vi "nanocal -- nuclear schottky goodness gradient.vi"(0 "zeta":dbl(slide)=0.23496699999999998 min=0.0 max=0.3 step=1e-06 scale=0.01..10.0 scale format="%#_3p", 1 "T1":dbl(slide)=0.26762 min=0.0 max=0.3 step=1e-06 scale=0.001..10.0 scale format="%#_3p", 2 "tauS":dbl(slide)=0.24445899999999998 min=0.0 max=0.3 step=1e-06 scale=0.001..10.0 scale format="%#_3p", 3 "tauN":dbl(slide)=2.349673 min=0.0 max=0.3 step=1e-06 scale=0.001..10.0 scale format="%#_3p", 4 "tauC":dbl(slide)=0.0059759999999999995 min=0.0 max=0.3 step=1e-06 scale=0.001..10.0 scale format="%#_3p", 5 "kappa0":dbl(slide)=5.58e-10 min=0.0 max=0.3 step=1e-12 scale=1e-10..1e-06 scale format="%#_3p", 6 "action":T1, 7 "Freq  (rad/sec)":dbl[](array[numeric])=[32012.991918577427, 32390.261658505893, 32466.39798177853, 32499.14340521798, 32517.39286113775, 32529.046092051318, 32537.14525712326, 32543.111142615544, 32547.696343954158, 32551.33675949651, 32554.302325209504, 32556.769142360055, 32558.856995237307, 32560.650202739795, 32562.209843476354, 32563.58125099723, 32564.7987833122, 32565.88895894197, 32566.872575330308, 32567.766175404246, 32568.583086316496, 32569.334166794306, 32570.02835688638, 32570.673085530187, 32571.274580490695, 32571.838104118455, 32572.36813539066, 32572.868514009202, 32573.342552524307, 32573.793126289274, 32574.222746575288, 32574.633618125405, 32575.027687968828, 32575.40668442971, 32575.772149741057, 32576.12546690325, 32576.467883345118, 32576.800529469096, 32577.124435064776, 32577.440543590797, 32577.749724325146, 32578.052781957467, 32578.35046682089, 32578.643482565894, 32578.932492128843, 32579.218126471686, 32579.500987779396, 32579.781656707495, 32580.06069600583, 32580.338656060805, 32580.616078519142, 32580.89350097748, 32581.171461032456, 32581.45050033079, 32581.73116925889, 32582.0140305666, 32582.29966469628, 32582.58867447239, 32582.88169000423, 32583.179375080817, 32583.48243271314, 32583.791613234323, 32584.10772197351, 32584.43162756919, 32584.764273480003, 32585.106690135035, 32585.460007297228, 32585.825472395412, 32586.204468856296, 32586.59853891288, 32587.009410462997, 32587.439030535847, 32587.889604513977, 32588.363642815923, 32588.86402143446, 32589.39405291983, 32589.957576334426, 32590.559071508098, 32591.203800151903, 32591.897990030815, 32592.64907072179, 32593.46598163404, 32594.359581707977, 32595.343197883154, 32596.433373726086, 32597.650906041054, 32599.022313348767, 32600.58195429849, 32602.375161800977, 32604.46301467823, 32606.929831615616, 32609.895397541775, 32613.535812870963, 32618.12101442274, 32624.086899701866, 32632.186064986967, 32643.839295900536, 32662.088751820305, 32694.834175046595, 32770.97049853239], 8 "dlogstep":dbl=0.0001 format="%#_13g", 9 "Voltage out (V)":cdb[](array[numeric])=[1.7183506006211996e-05-0.0001154032788780638i, 1.7124360968751133e-05-0.0001154114779288915i, 1.7049104347380084e-05-0.00011541542942613611i, 1.700437896335042e-05-0.00011541749156201827i, 1.6984579723285106e-05-0.00011542204741013496i, 1.702277369054923e-05-0.00011543195548892015i, 1.713094025845651e-05-0.00011543928112855599i, 1.734249707866828e-05-0.00011543960094139092i, 1.768320429215342e-05-0.0001154245402225022i, 1.8195281152538477e-05-0.00011538335923575508i, 1.8917228661806973e-05-0.00011530288392402138i, 1.9897834564883332e-05-0.00011516640933089982i, 2.154104046962704e-05-0.0001148906117047364i, 2.3247799321765792e-05-0.00011455940834964969i, 2.5364678450551808e-05-0.00011410149936074356i, 2.8645788781885885e-05-0.00011331572480450341i, 3.204749554800641e-05-0.00011242961468546203i, 3.783559691555022e-05-0.00011080033368711338i, 4.245015867332296e-05-0.00010941815048749576i, 4.909131821431355e-05-0.0001073312840925185i, 5.511821898441184e-05-0.00010535829212367013i, 6.178843506022867e-05-0.00010310289174359778i, 7.1079604965352e-05-9.985157907779013e-05i, 7.922304381453334e-05-9.690255343156676e-05i, 8.814778883893872e-05-9.35627973091444e-05i, 9.806709148886077e-05-8.971246458508318e-05i, 0.00011119043245647465-8.437841897470898e-05i, 0.00012253184919712196-7.953180105990741e-05i, 0.00013777724317049346-7.26422052575784e-05i, 0.0001508081004573332-6.638511645494567e-05i, 0.00016547294918783876-5.890291826790314e-05i, 0.00018003847596605868-5.097295421607585e-05i, 0.00019518361086534857-4.2160672625888326e-05i, 0.00021134179818259658-3.207632261667366e-05i, 0.0002372041782935464-1.434566976209705e-05i, 0.00025518143132024254-7.65423157605567e-07i, 0.0002835129702467886+2.297908707067173e-05i, 0.0003060118087631287+4.414715126576145e-05i, 0.00032860772064336976+6.780161699354136e-05i, 0.0003492674091322389+9.188627597766353e-05i, 0.00037498324855458583+0.0001258445655672888i, 0.00040021078021115026+0.00016463936720210011i, 0.00041969942568205823+0.0001996255883353531i, 0.00044367338947118773+0.00025154867300893595i, 0.0004634793607238068+0.0003068834938295352i, 0.00047921028781215815+0.00036805191402776324i, 0.0004880906353641744+0.00042166295770603194i, 0.0004932212623741357+0.0004947057496862386i, 0.000491476456593048+0.0005562791342814882i, 0.000480893803992059+0.0006363872629062725i, 0.0004535995818650303+0.0007373086546111893i, 0.000417087772881063+0.0008226852134031236i, 0.0003564148692854789+0.0009214817173403453i, 0.0003049201646356487+0.0009841224100520793i, 0.00021260191240459413+0.0010684135492785532i, 0.00011714858948470126+0.001130293664798013i, 1.675457544365132e-05+0.0011752384955043165i, -6.8674075405897e-05+0.0012001399159748158i, -0.000156473047607305+0.0012143601357779102i, -0.00026709373934749337+0.0012167952520739987i, -0.0003544271565676041+0.001206585218500233i, -0.00047937600197311275+0.0011721904461218277i, -0.0006086290582260493+0.0011080263068835828i, -0.0007031877411848573+0.0010369948237613604i, -0.0007564526901441745+0.0009845652865779295i, -0.000802489180995596+0.0009292050493656664i, -0.0008414596018105983+0.0008721985101652608i, -0.0008809346482248761+0.0008000538120167723i, -0.0009073902840241921+0.0007382113118499092i, -0.0009264953054508651+0.000680980624166274i, -0.0009405659412141811+0.0006247883223244968i, -0.000951649722530156+0.0005564170049287236i, -0.0009557485581057351+0.0005027508202624884i, -0.0009558464741053665+0.0004515634249715623i, -0.0009509110176922098+0.0003899637122391104i, -0.0009411315169847015+0.00033238768338539245i, -0.0009303400913929496+0.0002890952314710416i, -0.0009171113529290538+0.00024772942260094455i, -0.0009022111527275027+0.00020961974320628598i, -0.0008813746494947608+0.00016554205395646727i, -0.0008581837971946129+0.00012481593212717478i, -0.0008372063466683705+9.328565348151487e-05i, -0.0008165626610594428+6.595676342721183e-05i, -0.0007901155435838691+3.51376371228606e-05i, -0.0007682834352800848+1.2585785624721776e-05i, -0.000746231015527196-7.956667433689733e-06i, -0.0007238798463130141-2.6771164006128246e-05i, -0.0007015567569177018-4.3779400880525094e-05i, -0.000679301954671598-5.9154880569231366e-05i, -0.0006572001413831251-7.301304884663801e-05i, -0.000629855254567978-8.838260380910578e-05i, -0.0006083942229188815-9.917719243438264e-05i, -0.0005768631156754208-0.00011317657292622015i, -0.0005562177438951648-0.00012121832857134644i, -0.0005359092039599222-0.00012831021292074535i, -0.0005145186443378148-0.00013494179211461784i, -0.0004951602053444319-0.00014023403510992087i, -0.00047624970229075174-0.00014478034103386663i, -0.0004577401041527736-0.00014865456703421655i, -0.00043519037796120065-0.00015262867452433312i], 10 "nymber of steps":i32=11) -> (14 "derivative":dbl format="%0.4f", 17 "goodness":dbl, 18 "log10goodness":dbl)   [LabVIEW 2020]
uses:
  3-lorentzian-heat-response action.ctl
  3-lorentzian-heat-response.vi
  3-lorentzian-heat-response.vi/142dd4c5-f9ed-c64b-bc14-a88e3e2c450a.vi
  <vilib>/Analysis/polynomials.llb/Multiply Polynomials.vi
  <vilib>/Analysis/polynomials.llb/Multiply Polynomials (DBL).vi
  <vilib>/Analysis/polynomials.llb/Polynomial Roots.vi
  <vilib>/Analysis/polynomials.llb/Polynomial Roots (DBL).vi
  <vilib>/Comparison/Less/Less Functor/Less Functor.lvclass
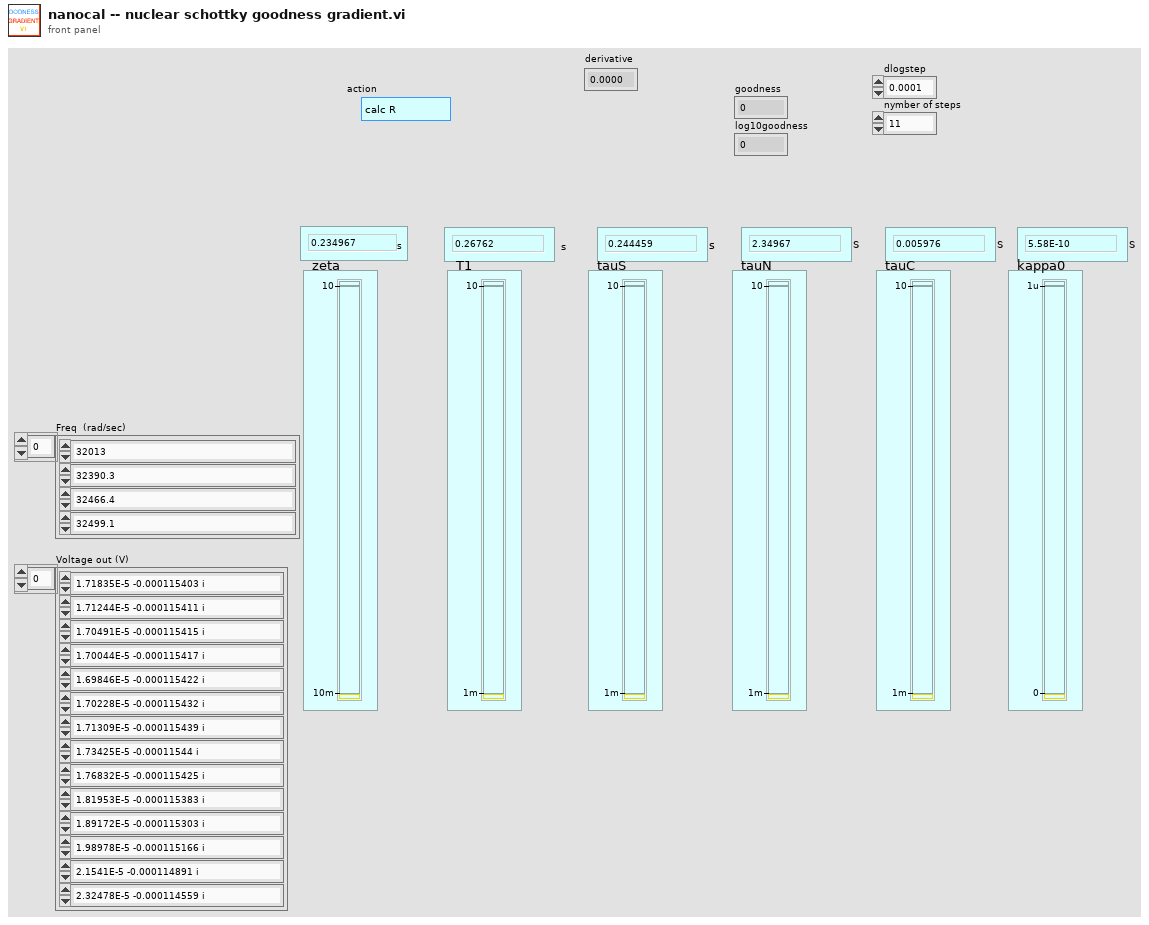
[diagram p1: front panel]
types:
  T1 = typedef "3-lorentzian-heat-response action.ctl" = enum16{"calc R", "create string", "calc m1m2m3", "dζ", "dT1", "dτS", "dτN", "dτC", "d-all", "dκ0"}
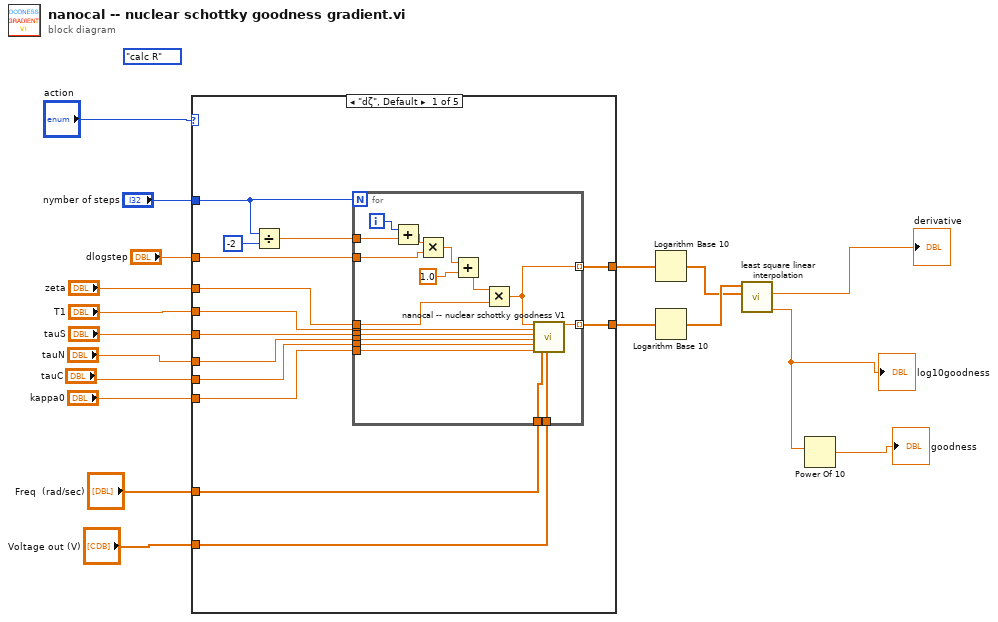
[diagram p0: block diagram]
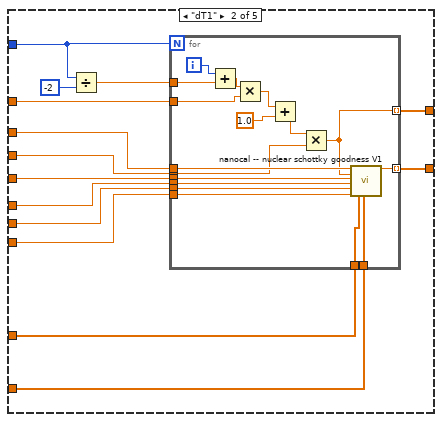
[diagram p2: hidden frame]
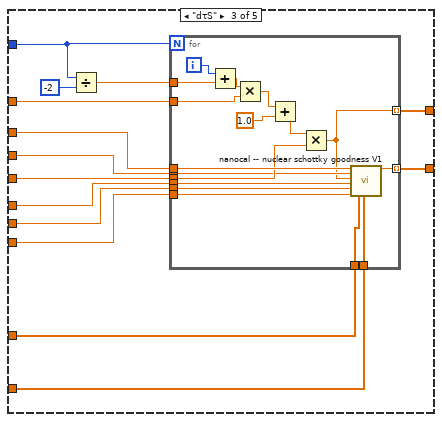
[diagram p3: hidden frame]
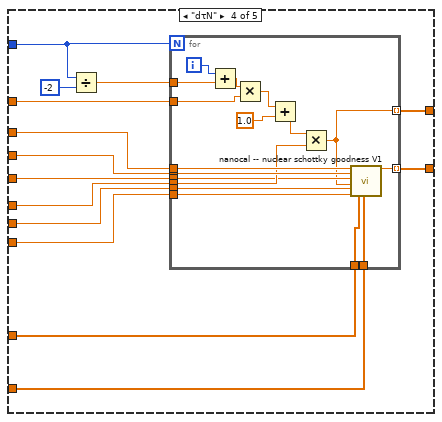
[diagram p4: hidden frame]
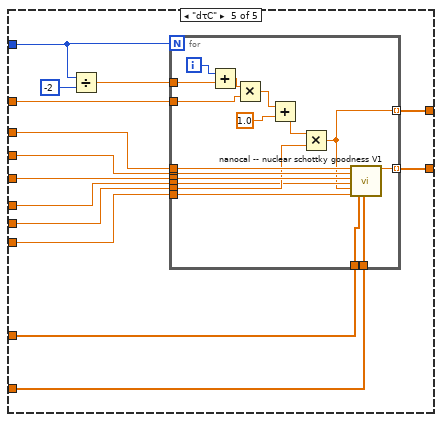
[diagram p5: hidden frame]
diagram:
  (unwired) 3-lorentzian-heat-response_action."calc R" ("action")
  n1 = case shown="\"dζ\", Default" "action" {
    tunnel: "T1" -> [w32 w63 w94 w125 w156]
    tunnel: "tauS" -> [w31 w62 w93 w124 w155]
    tunnel: "tauN" -> [w30 w61 w92 w123 w154]
    tunnel: "tauC" -> [w29 w60 w91 w122 w153]
    tunnel: [w28 w59 w90 w121 w152] -> w9
    tunnel: "Freq  (rad/sec)" -> [w27 w58 w89 w120 w151]
    tunnel: "Voltage out (V)" -> [w26 w57 w88 w119 w150]
    tunnel: "kappa0" -> [w24 w55 w86 w117 w148]
    tunnel: "zeta" -> [w25 w56 w87 w118 w149]
    tunnel: [w19 w50 w81 w112 w143] -> w10
    tunnel: "nymber of steps" -> [w21 w52 w83 w114 w145]
    tunnel: "dlogstep" -> [w20 w51 w82 w113 w144]
    frame "dζ", Default {
      n2 = Divide(x=w21, y=-2) -> (x/y=w22:dbl)
      n3 = for {
        N: w21 -> [_]
        tunnel: w32 -> [w49]
        tunnel: w31 -> [w48]
        tunnel: w30 -> [w47]
        tunnel: w29 -> [w46]
        tunnel: [w45] -> w28 mode=indexing
        tunnel: w27 -> [w44]
        tunnel: w26 -> [w43]
        tunnel: w25 -> [w35]
        tunnel: w24 -> [w42]
        tunnel: w22 -> [w40]
        tunnel: w20 -> [w36]
        tunnel: [w33] -> w19 mode=indexing
        i -> [w41]
        n4 = Add(x=w41, y=w40) -> (x+y=w39:dbl)
        n5 = Multiply(x=w39, y=w36) -> (x*y=w38:dbl)
        n6 = Add(x=w38, y=1.0) -> (x+y=w34:dbl)
        n7 = Multiply(x=w34, y=w35) -> (x*y=w33:dbl)
        n8 = call "nanocal -- nuclear schottky goodness V1.vi"("ζ"=w33, "T1"=w49, "τS"=w48, "τN"=w47, "τC"=w46, "κ0"=w42, "Freq out (rad/sec)"=w44, "Voltage out (V)"=w43) -> ("result"=w45:dbl)  [unwired: 11 in]
      }
    }
    frame "dT1" {
      n9 = Divide(x=w52, y=-2) -> (x/y=w53:dbl)
      n10 = for {
        N: w52 -> [_]
        tunnel: w63 -> [w65]
        tunnel: w62 -> [w80]
        tunnel: w61 -> [w79]
        tunnel: w60 -> [w78]
        tunnel: [w77] -> w59 mode=indexing
        tunnel: w58 -> [w76]
        tunnel: w57 -> [w75]
        tunnel: w56 -> [w66]
        tunnel: w55 -> [w74]
        tunnel: w53 -> [w72]
        tunnel: w51 -> [w68]
        tunnel: [w64] -> w50 mode=indexing
        i -> [w73]
        n11 = Add(x=w73, y=w72) -> (x+y=w71:dbl)
        n12 = Multiply(x=w71, y=w68) -> (x*y=w70:dbl)
        n13 = Add(x=w70, y=1.0) -> (x+y=w67:dbl)
        n14 = Multiply(x=w67, y=w65) -> (x*y=w64:dbl)
        n15 = call "nanocal -- nuclear schottky goodness V1.vi"("ζ"=w66, "T1"=w64, "τS"=w80, "τN"=w79, "τC"=w78, "κ0"=w74, "Freq out (rad/sec)"=w76, "Voltage out (V)"=w75) -> ("result"=w77:dbl)  [unwired: 11 in]
      }
    }
    frame "dτS" {
      n16 = Divide(x=w83, y=-2) -> (x/y=w84:dbl)
      n17 = for {
        N: w83 -> [_]
        tunnel: w94 -> [w96]
        tunnel: w93 -> [w97]
        tunnel: w92 -> [w111]
        tunnel: w91 -> [w110]
        tunnel: [w109] -> w90 mode=indexing
        tunnel: w89 -> [w108]
        tunnel: w88 -> [w107]
        tunnel: w87 -> [w98]
        tunnel: w86 -> [w106]
        tunnel: w84 -> [w104]
        tunnel: w82 -> [w100]
        tunnel: [w95] -> w81 mode=indexing
        i -> [w105]
        n18 = Add(x=w105, y=w104) -> (x+y=w103:dbl)
        n19 = Multiply(x=w103, y=w100) -> (x*y=w102:dbl)
        n20 = Add(x=w102, y=1.0) -> (x+y=w99:dbl)
        n21 = Multiply(x=w99, y=w97) -> (x*y=w95:dbl)
        n22 = call "nanocal -- nuclear schottky goodness V1.vi"("ζ"=w98, "T1"=w96, "τS"=w95, "τN"=w111, "τC"=w110, "κ0"=w106, "Freq out (rad/sec)"=w108, "Voltage out (V)"=w107) -> ("result"=w109:dbl)  [unwired: 11 in]
      }
    }
    frame "dτN" {
      n23 = Divide(x=w114, y=-2) -> (x/y=w115:dbl)
      n24 = for {
        N: w114 -> [_]
        tunnel: w125 -> [w129]
        tunnel: w124 -> [w127]
        tunnel: w123 -> [w128]
        tunnel: w122 -> [w142]
        tunnel: [w141] -> w121 mode=indexing
        tunnel: w120 -> [w140]
        tunnel: w119 -> [w139]
        tunnel: w118 -> [w130]
        tunnel: w117 -> [w138]
        tunnel: w115 -> [w136]
        tunnel: w113 -> [w132]
        tunnel: [w126] -> w112 mode=indexing
        i -> [w137]
        n25 = Add(x=w137, y=w136) -> (x+y=w135:dbl)
        n26 = Multiply(x=w135, y=w132) -> (x*y=w134:dbl)
        n27 = Add(x=w134, y=1.0) -> (x+y=w131:dbl)
        n28 = Multiply(x=w131, y=w128) -> (x*y=w126:dbl)
        n29 = call "nanocal -- nuclear schottky goodness V1.vi"("ζ"=w130, "T1"=w129, "τS"=w127, "τN"=w126, "τC"=w142, "κ0"=w138, "Freq out (rad/sec)"=w140, "Voltage out (V)"=w139) -> ("result"=w141:dbl)  [unwired: 11 in]
      }
    }
    frame "dτC" {
      n30 = Divide(x=w145, y=-2) -> (x/y=w146:dbl)
      n31 = for {
        N: w145 -> [_]
        tunnel: w156 -> [w161]
        tunnel: w155 -> [w160]
        tunnel: w154 -> [w158]
        tunnel: w153 -> [w159]
        tunnel: [w173] -> w152 mode=indexing
        tunnel: w151 -> [w172]
        tunnel: w150 -> [w171]
        tunnel: w149 -> [w162]
        tunnel: w148 -> [w170]
        tunnel: w146 -> [w168]
        tunnel: w144 -> [w164]
        tunnel: [w157] -> w143 mode=indexing
        i -> [w169]
        n32 = Add(x=w169, y=w168) -> (x+y=w167:dbl)
        n33 = Multiply(x=w167, y=w164) -> (x*y=w166:dbl)
        n34 = Add(x=w166, y=1.0) -> (x+y=w163:dbl)
        n35 = Multiply(x=w163, y=w159) -> (x*y=w157:dbl)
        n36 = call "nanocal -- nuclear schottky goodness V1.vi"("ζ"=w162, "T1"=w161, "τS"=w160, "τN"=w158, "τC"=w157, "κ0"=w170, "Freq out (rad/sec)"=w172, "Voltage out (V)"=w171) -> ("result"=w173:dbl)  [unwired: 11 in]
      }
    }
  }
  n37 = Logarithm Base 10(1:w10) -> (0:w4:dbl[])
  n38 = Logarithm Base 10(1:w9) -> (0:w5:dbl[])
  n39 = call "least square linear interpolation.vi"("X"=w4, "Y"=w5) -> ("mean Y"=w2:dbl, "slope"=→"derivative":dbl)  [unwired: 6 in, 2 out]
  "log10goodness" <- w2
  n40 = Power Of 10(x=w2) -> (10^x=→"goodness":dbl)
